vi "素材.vi"() -> ()   [LabVIEW 2018]
uses:
  <vilib>/measure/NI_MABase.lvlib
  <vilib>/measure/NI_MAPro.lvlib
panel:
  out "波形图 2":waveform(dbl)(graph)
  in  "sampling info 3":cluster{"Fs":dbl, "#s":dbl}={"Fs"=1000.0, "#s"=1000.0} caption="采样信息" {"Fs" format="%.2p"}
  in  "amplitude 3":dbl=3.0 caption="幅值3" format="%0.2f"
  in  "amplitude 2":dbl=2.0 caption="幅值2" format="%0.2f"
  in  "amplitude 1":dbl=4.0 caption="幅值1" format="%0.2f"
  in  "phase 3":dbl=135.0 caption="相位3" format="%0.2f"
  in  "phase 2":dbl=90.0 caption="相位2" format="%0.2f"
  in  "phase 1":dbl caption="相位1" format="%0.2f"
  in  "频率":dbl
  in  "sampling info 2":cluster{"Fs":dbl, "#s":dbl}={"Fs"=1000.0, "#s"=1000.0} caption="采样信息" {"Fs" format="%.2p"}
  in  "amplitude 2":dbl=1.0 caption="幅值" format="%.2p"
  out "波形图":waveform(dbl)(graph)
  in  "frequency":dbl=10.0 caption="频率" format="%0.2p"
  in  "amplitude":dbl=1.0 caption="幅值" format="%0.2p"
  in  "phase":dbl caption="相位" format="%.2p"
  in  "reset signal":bool caption="重置信号"
  in  "sampling info":cluster{"Fs":dbl, "#s":dbl}={"Fs"=1000.0, "#s"=1000.0} caption="采样信息" {"Fs" format="%.2p"}
  in  "offset":dbl caption="偏移量" format="%0.2p"
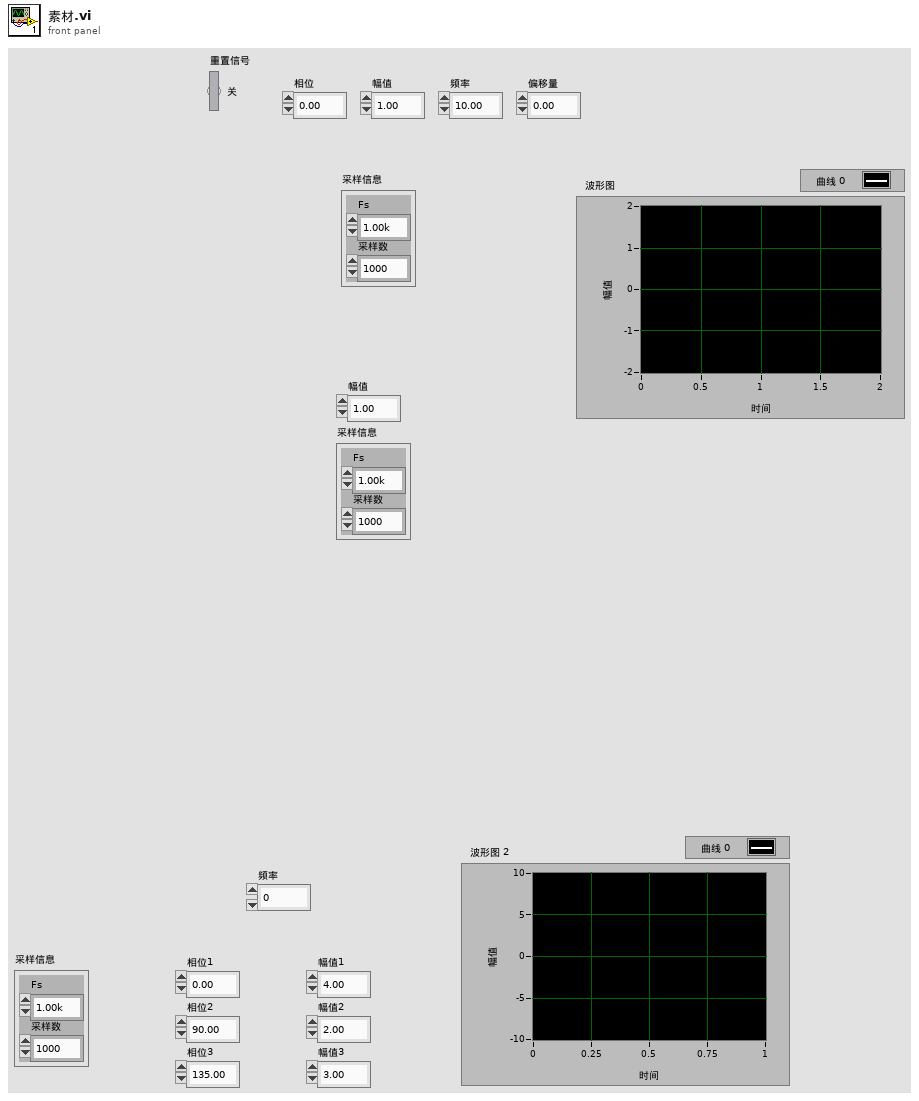
[diagram p1: front panel]
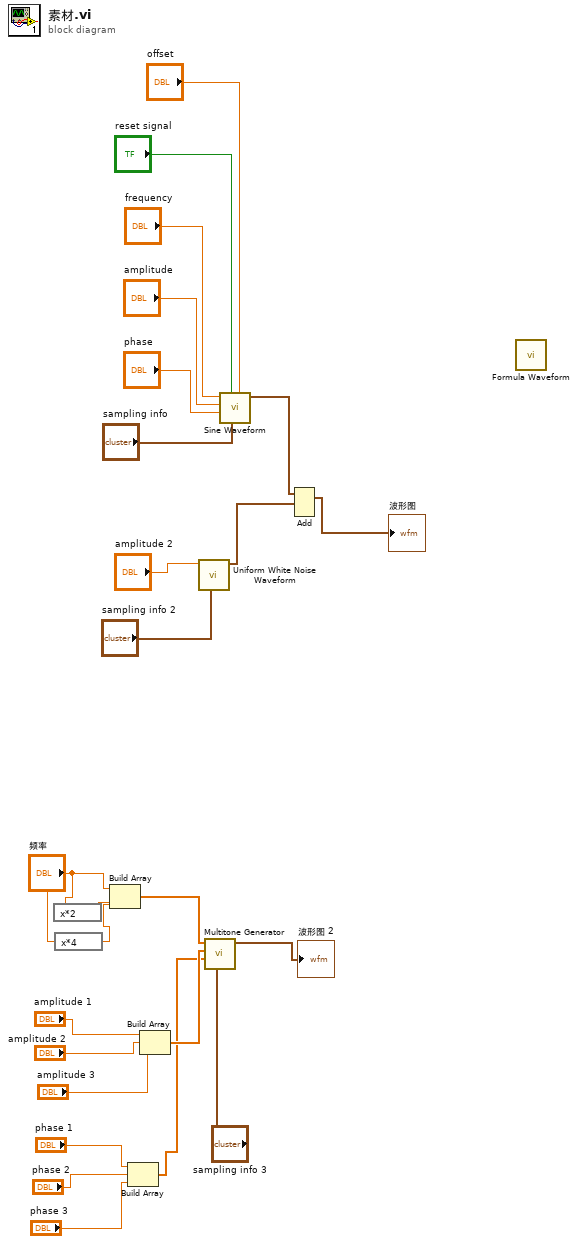
[diagram p0: block diagram]
diagram:
  n1 = expression code="x*2"("频率") -> (w14:dbl)
  n2 = expression code="x*4"("频率") -> (w13:dbl)
  n3 = Build Array("频率", w14, w13) -> (w11:dbl[])
  n4 = Build Array("phase 1", "phase 2", "phase 3") -> (w3:dbl[])
  n5 = Build Array("amplitude 1", "amplitude 2", "amplitude 3") -> (w4:dbl[])
  n6 = call <vilib>:"Uniform White Noise Waveform.vi"("sampling info"="sampling info 2", "amplitude"="amplitude 2") -> ("signal out"=w17:waveform(dbl))  [unwired: 8 in, 1 out]
  n7 = call <vilib>:"Multitone Generator.vi"("sampling info"="sampling info 3", "tone phases"=w3, "tone amplitudes"=w4, "tone frequencies"=w11) -> ("signal out"=→"波形图 2":waveform(dbl))  [unwired: 4 in, 3 out]
  n8 = call <vilib>:"Sine Waveform.vi"("offset"="offset", "sampling info"="sampling info", "reset signal"="reset signal", "phase"="phase", "amplitude"="amplitude", "frequency"="frequency") -> ("signal out"=w16:waveform(dbl))  [unwired: 4 in, 1 out]
  n9 = Add(1:w17, 2:w16) -> (0:→"波形图":waveform(dbl))  [unwired: 1 in, 1 out]
  n10 = call <vilib>:"Formula Waveform.vi"() -> ()  [unwired: 10 in, 2 out]
